vi "SYST_DATE-TIME.vi"(0 "Session In":refnum<visa-resource-name>, 11 "error in":errorcluster) -> (2 "Date/Time(str)":string, 3 "timestamp":timestamp format="%<%H:%M:%S\n%d/%m/%Y>T", 4 "Session Out":refnum<visa-resource-name>, 15 "error out":errorcluster)   [LabVIEW 2018]
panel:
  out "date string":string
  out "time string":string
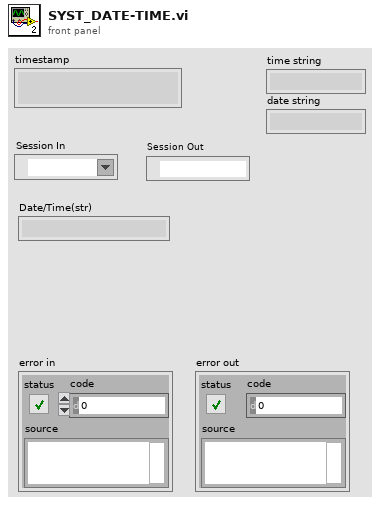
[diagram p1: front panel]
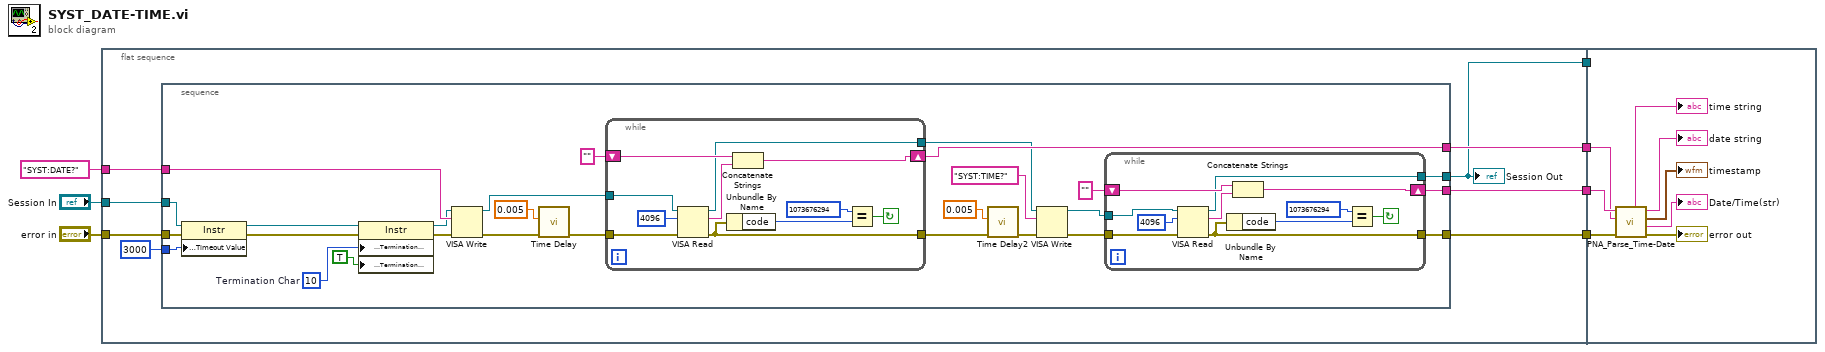
[diagram p0: block diagram]
diagram:
  n1 = flat-sequence {
    tunnel: "SYST:DATE?" ("Rcmd") -> [w15]
    tunnel: [w14] -> w6
    tunnel: [w13] -> w5
    tunnel: [w11] -> w4
    tunnel: [w10] -> w3
    tunnel: "Session In" -> [w9]
    tunnel: "error in" -> [w8]
    tunnel: w6 -> [w71]
    tunnel: w5 -> [_]
    tunnel: w4 -> [w72]
    tunnel: w3 -> [w70]
    frame #0 {
      n2 = stacked-sequence {
        tunnel: [w27] -> w13
        tunnel: [w42] -> w14
        tunnel: u32 3000 ("Timeout") -> [w35]
        tunnel: w8 -> [w34]
        tunnel: w15 -> [w41]
        tunnel: w9 -> [w36]
        tunnel: [w25] -> w11
        tunnel: [w24] -> w10
        frame #0 {
          w38 = u8 10  # Termination Char
          n3 = property class="Instr"(reference=w36, error in=w34, "General Settings:Timeout Value"=w35) -> (reference out=w39:refnum<visa-resource-name>, error out=w37:errorcluster)
          n4 = property class="Instr"(reference=w39, error in=w37, "Message Based Settings:Termination Character"=w38, "Message Based Settings:Termination Character Enable"=TRUE ("enable")) -> (reference out=w33:refnum<visa-resource-name>, error out=w32:errorcluster)
          n5 = VISA Write(VISA resource name=w33, write buffer=w41, error in (no error)=w32) -> (VISA resource name out=w31:refnum<visa-resource-name>, error out=w20:errorcluster)  [unwired: 1 out]
          n6 = call "Time Delay"("error in (no error)"=w20, "Delay Time (s)"=0.005) -> ("error out"=w21:errorcluster)  [unwired: 9 in]
          n7 = while {
            tunnel: w31 -> [w61]
            shift-right: [w55] -> w42
            shift-left: "" -> [w60]
            tunnel: w21 -> [w58]
            tunnel: [w57] -> w17
            tunnel: [w54] -> w29
            stop <- w56 continue-if-true
            n8 = VISA Read(VISA resource name=w61, byte count=u32 4096 ("byte count (0)"), error in (no error)=w58) -> (VISA resource name out=w54:refnum<visa-resource-name>, read buffer=w59:string, error out=w57:errorcluster)  [unwired: 1 out]
            n9 = Unbundle By Name(w57) -> ("code"=w63:i32)
            n10 = Concatenate Strings(w60, w59) -> (w55:string)
            n11 = Equal?(x=1073676294, y=w63) -> (x = y?=w56:bool)
          }
          n12 = call "Time Delay2"("error in (no error)"=w17, "Delay Time (s)"=0.005) -> ("error out"=w18:errorcluster)  [unwired: 9 in]
          n13 = VISA Write(VISA resource name=w29, write buffer="SYST:TIME?", error in (no error)=w18) -> (VISA resource name out=w28:refnum<visa-resource-name>, error out=w22:errorcluster)  [unwired: 1 out]
          n14 = while {
            tunnel: w28 -> [w50]
            shift-right: [w44] -> w25
            shift-left: "" -> [w49]
            tunnel: w22 -> [w47]
            tunnel: [w46] -> w24
            tunnel: [w43] -> w27
            stop <- w45 continue-if-true
            n15 = VISA Read(VISA resource name=w50, byte count=u32 4096 ("byte count (0)"), error in (no error)=w47) -> (VISA resource name out=w43:refnum<visa-resource-name>, read buffer=w48:string, error out=w46:errorcluster)  [unwired: 1 out]
            n16 = Unbundle By Name(w46) -> ("code"=w52:i32)
            n17 = Concatenate Strings(w49, w48) -> (w44:string)
            n18 = Equal?(x=1073676294, y=w52) -> (x = y?=w45:bool)
          }
        }
      }
      "Session Out" <- w13
    }
    frame #1 {
      n19 = call "PNA_Parse_Time-Date.vi"("error in (no error)"=w70, "SYST:DATE (IN)"=w71, "SYST:TIME (IN)"=w72) -> ("error out"=→"error out":errorcluster, "Time/Date Out (Str)"=→"Date/Time(str)":string, "Time Stamp"=→"timestamp":timestamp, "Date Out (str)"=→"date string":string, "Time Out (str)"=→"time string":string)  [unwired: 4 in]
    }
  }
